vi "test_popup.vi"(9 "value":dbl, 10 "config":T2={"hardware"=enum."microwaves (GHz)", "options"="", "repeats"=1, "loops"=1, "VISA"="COM9", "override_VISA"=FALSE} {"loops" min=1; "repeats" min=1}, 11 "generic settings":T1={"generic cmd"="", "upper_limit"=5.0, "lower limit"=0.05, "format"="%#.8g"} {"upper_limit" format="%#_13g"}) -> (3 "cancelled":bool)   [LabVIEW 2017, in "tools.lvlib"]
uses:
  tools.lvlib
  core/var_config.ctl
  ctrl/var_list.ctl
  core/generic_config.ctl
panel:
  in  "Cancel":bool
  in  "Test":bool
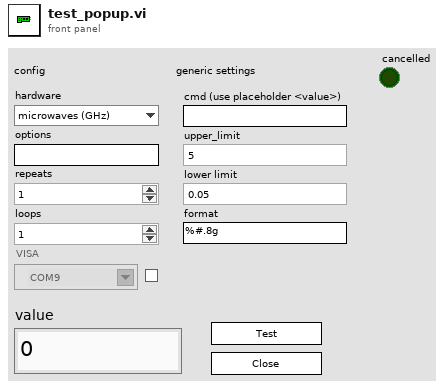
[diagram p1: front panel]
types:
  T1 = typedef "tools.lvlib/generic_config.ctl" = cluster{"generic cmd":string, "upper_limit":dbl, "lower limit":dbl, "format":string}
  T2 = typedef "tools.lvlib/var_config.ctl" = cluster{"hardware":T3, "options":string, "repeats":i32, "loops":i32, "VISA":refnum<visa-resource-name>, "override_VISA":bool}
  T3 = typedef "var_list.ctl" = enum16{"none", "AO voltage (V)", "delay (s)", "generic", "microwaves (GHz)", "radiant (nm)", "radiant thg (nm)", "sirah (nm)", "sirah_shg (nm)", "tenma voltage (V)", "wait (s)", "wf_freq (Hz)", "wf_amp (V)", "wf_amp_multi (V)", "wf_offset (V)", "wf_low_level (V)", "wf_high_level (V)", "wf_period (s)", "wf_pulse_width (s)", "wf_sample_rate (Sa/s)", "wf_multi_amp", "wf_multi_freq", "wf_arb_4chan", "WS7 setpoint (nm)"}
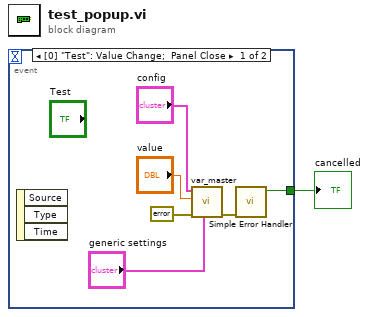
[diagram p0: block diagram]
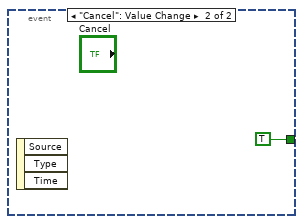
[diagram p2: hidden frame]
diagram:
  n1 = event shown="[0] \"Test\": Value Change;  Panel Close" {
    selector: _ -> [_ _]
    dyn-events: _ -> [_ _]
    timeout: _ -> [_ _]
    tunnel: [w7 TRUE ("Cancel")] -> w1
    event "Test": Value Change; Panel Close {
      n2 = event-data() -> ()  [unwired: 1 in, 3 out]
      n3 = call "var_master.vi"("generic settings"="generic settings", "error IN"=errorcluster {"status"=FALSE, "code"=0, "source"=""} ("error out"), "value IN"="value", "config"="config") -> ("error OUT"=w3:errorcluster)  [unwired: 6 in, 1 out]
      n4 = call <vilib>:"Simple Error Handler.vi"("error in (no error)"=w3) -> ("error?"=w7:bool)  [unwired: 4 in, 4 out]
    }
    event "Cancel": Value Change {
      n5 = event-data() -> ()  [unwired: 1 in, 3 out]
    }
  }
  "cancelled" <- w1
